vi "CreatePublicEvents.vi"(8 "error in (no error)":errorcluster, 11 "DAQmx":refnum<class "DAQmx.lvclass">) -> (0 "error out":errorcluster, 3 "DAQmx out":refnum<class "DAQmx.lvclass">)   [LabVIEW 2019, in "DAQmx.lvclass"]
uses:
  DAQmx.lvclass
  typedefs/DAQmx.Status--enum.ctl
  typedefs/DeviceInfo--Cluster.ctl
  typedefs/DAQ.Config.AO--Cluster--Array.ctl
  typedefs/DAQ.Config.AO--Cluster.ctl
  typedefs/DAQ.Config.AO.Range--enum.ctl
  typedefs/DAQ.Config.Device Type--enum.ctl
  typedefs/DAQ.Config.AI--Cluster--Array.ctl
  typedefs/DAQ.Config.AI--Cluster.ctl
  typedefs/DAQ.Config.AI.Coupling--enum.ctl
  typedefs/DAQ.Config.AI.Range--enum.ctl
  typedefs/DAQ.Config.Timing--Cluster.ctl
  typedefs/DAQ.Config.Timing.Sampling--Cluster.ctl
  typedefs/DAQ.Config.Timing.Fs Mode--enum.ctl
  typedefs/DAQ.Calibration--Cluster--Array.ctl
  typedefs/DAQ.Calibration--Cluster.ctl
  DAQmx.lvclass/DAQmx.ctl
  <vilib>/JKI/JKI SMO/SMO/SMO.lvclass
panel:
  # "For instructions on how to use the JKI State Machine Objects, examples and video tutorials, visit:\nhttp://jki.net/state-machine-objects/\n\nJKI State Machine Objects™\nhttp://jki.net/state-machine-objects/\nCopyright (C) 2005-2015, JKI <info@jki.net>\nALL RIGHTS RESERVED"
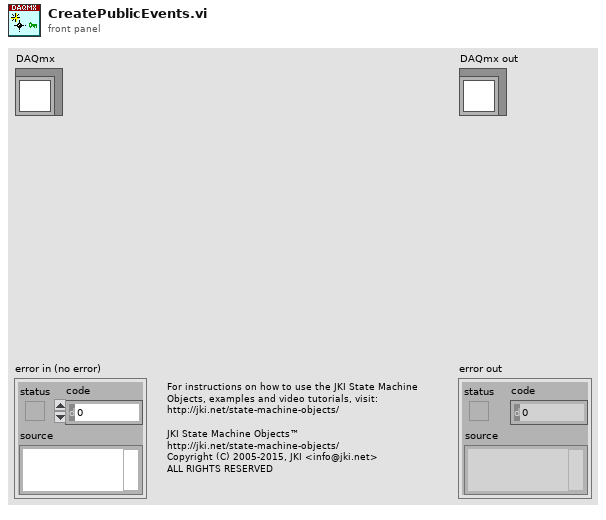
[diagram p1: front panel]
types:
  T1 = typedef "DAQmx.lvclass/DAQ.Calibration--Cluster--Array.ctl" = T2[]
  T2 = typedef "DAQmx.lvclass/DAQ.Calibration--Cluster.ctl" = cluster{"Active Device":string, "SelfCal.LastDate/Time":dbl, "SelfCal.LastTemp":dbl, "DevTemp":dbl, "calibration due?":bool}
  T3 = typedef "DAQmx.lvclass/DAQ.Config.Timing--Cluster.ctl" = cluster{"Sampling":T4, "sample mode":i32, "FsMode":T5, "Fs Multiplier":dbl, "Refresh Rate (Hz)":dbl, "Decimation.PreDSP":i32, "Decimation.PostDSP":i32, "Fs.Output":dbl}
  T4 = typedef "DAQmx.lvclass/DAQ.Config.Timing.Sampling--Cluster.ctl" = cluster{"Fs":dbl, "#s":i32}
  T5 = typedef "DAQmx.lvclass/DAQ.Config.Timing.Fs Mode--enum.ctl" = enum16{"Manual", "Auto Fs", "Max Fs"}
  T6 = typedef "DAQmx.lvclass/DAQ.Config.AI--Cluster--Array.ctl" = T7[]
  T7 = typedef "DAQmx.lvclass/DAQ.Config.AI--Cluster.ctl" = cluster{"Channels":tag, "Coupling":T8, "Range":T9, "input terminal configuration":i32, "Type":T10}
  T8 = typedef "DAQmx.lvclass/DAQ.Config.AI.Coupling--enum.ctl" = u16
  T9 = typedef "DAQmx.lvclass/DAQ.Config.AI.Range--enum.ctl" = enum16{"±0.316", "±1.00", "±3.16", "±10.0", "±31.6", "±42.4", ""}
  T10 = typedef "DAQmx.lvclass/DAQ.Config.Device Type--enum.ctl" = enum16{"None", "USB-4431", "PXI-446x"}
  T11 = typedef "DAQmx.lvclass/DAQ.Config.AO--Cluster--Array.ctl" = T12[]
  T12 = typedef "DAQmx.lvclass/DAQ.Config.AO--Cluster.ctl" = cluster{"Channels":tag, "Range":T13, "output terminal configuration":i32, "Type":T10}
  T13 = typedef "DAQmx.lvclass/DAQ.Config.AO.Range--enum.ctl" = enum16{"±0.1", "±1.0", "±10.0", ""}
  T14 = typedef "DAQmx.lvclass/DeviceInfo--Cluster.ctl" = cluster{"DeviceName":string, "DevIsSimulated":bool, "DeviceSerialNumber":u32, "ProductType":string, "ProductCategory":i32, "ProductNumber":u32, "ChassisNumber":u32, "SlotNumber":u32, "ChassisName":string, "ChassisSerialNumber":u32}
  T15 = typedef "DAQmx.lvclass/DAQmx.Status--enum.ctl" = enum16{"idle", "calibrating", "configuring", "creating", "created", "starting", "started", "stopping", "stopped", "clearing"}
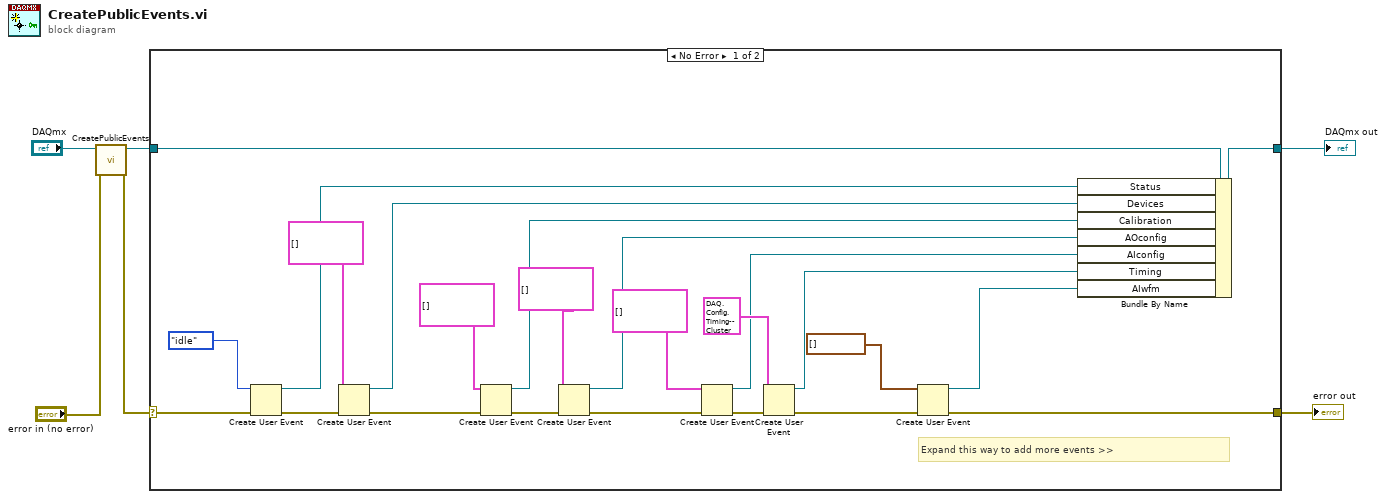
[diagram p0: block diagram]
diagram:
  n1 = call-parent "CreatePublicEvents.vi"("error in (no error)"="error in (no error)", "SMO"="DAQmx") -> ("error out"=w1:errorcluster, "SMO out"=w5:refnum<class "DAQmx.lvclass">)  [unwired: 8 in]
  n2 = case shown="No Error" w1 {
    selector: w1 -> [w26 w32]
    tunnel: [w29 w32] -> w3
    tunnel: [w30 w31] -> w4
    tunnel: w5 -> [w23 w31]
    frame No Error {
      # "Expand this way to add more events >>"
      n3 = Create User Event(user event datatype=DAQmx.Status--enum."idle" ("Status"), error in=w26) -> (user event=w24:refnum<user-event>, error out=w15:errorcluster)
      n4 = Create User Event(user event datatype=T14[] [] ("event data"), error in=w15) -> (user event=w16:refnum<user-event>, error out=w10:errorcluster)
      n5 = Create User Event(user event datatype=T1 [] ("Calibration"), error in=w10) -> (user event=w7:refnum<user-event>, error out=w9:errorcluster)
      n6 = Create User Event(user event datatype=T11 [] ("event data"), error in=w9) -> (user event=w17:refnum<user-event>, error out=w14:errorcluster)
      n7 = Create User Event(user event datatype=T6 [] ("event data"), error in=w14) -> (user event=w11:refnum<user-event>, error out=w13:errorcluster)
      n8 = Create User Event(user event datatype=T3 {"Sampling"={"Fs"=1000.0, "#s"=128}, "sample mode"=10123, "FsMode"=enum."Manual", "Fs Multiplier"=1.0, "Refresh Rate (Hz)"=10.0, "Decimation.PreDSP"=1, "Decimation.PostDSP"=1, "Fs.Output"=204789.0} ("event data"), error in=w13) -> (user event=w18:refnum<user-event>, error out=w12:errorcluster)
      n9 = Create User Event(user event datatype=waveform(dbl)[] [] ("Waveform"), error in=w12) -> (user event=w25:refnum<user-event>, error out=w29:errorcluster)
      n10 = Bundle By Name(cluster=w23, "Status"=w24, "Devices"=w16, "Calibration"=w7, "AOconfig"=w17, "AIconfig"=w11, "Timing"=w18, "AIwfm"=w25) -> (w30:refnum<class "DAQmx.lvclass">)
    }
    frame Error {
    }
  }
  "error out" <- w3
  "DAQmx out" <- w4
